vi "Set Trigger Pulse Width Ns.vi"(10 "up_ns":i32, 11 "down_ns":i32) -> ()   [LabVIEW 2021, in "vmmso.lvlib"]
doc: "DLL_API void WINAPI SetTriggerPulseWidthNs(int down_ns, int up_ns);"
uses:
  vmmso.lvlib
  vmmso.dll
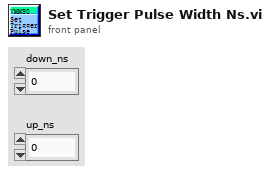
[diagram p1: front panel]
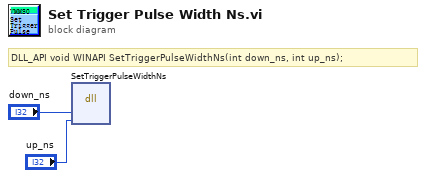
[diagram p0: block diagram]
diagram:
  # "DLL_API void WINAPI SetTriggerPulseWidthNs(int down_ns, int up_ns);"
  n1 = dll-call lib="D:/labviewdemo/LabviewDemo 21/vmmso/vmmso.*" fn="SetTriggerPulseWidthNs"("down_ns"="down_ns", "up_ns"="up_ns") -> ()  [unwired: 6 in, 2 out]
